vi "ttm_creep_poller.vi"() -> ()   [LabVIEW 2011]
doc: "This is the sample data playback waveform and data logging example program. Sample data points are generated using MX Sample Data Array Generator.vi. You will need to replace this VI with your own code. New sample data is sent to the controller each time a status message is recieved from the controller that the next random buffer is running.\nThis program also shows you how to use Active X events. These are used to notify the program when a data buffer is ready for collection and when to load a new buffer of sample data points. Two separate event queues are used: one for data logging and the other for general status, such as when a sample data point buffer can be sent to the controller. Each event handler must run in parallel loops as execution passes to MX Handle Status Change Event.vi and MX Handle Data Ready Event.vi and will not come out of them until an event is received from the console program. When modifiying this example for your own use you may want to setup a third loop to be doing other processing, or you could add code to manipulate the data buffer in the data monitoring loop."
panel:
  out "Number of points":i32=1000
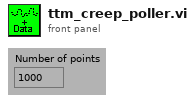
[diagram p1: front panel]
types:
  T1 = cluster{"Data Sample Format (0)":i8, "Loop code (2)":i8, "Target Amplitude (32767)":i16, "Playback rate":dbl, "Playback Scale":dbl[], "Envelope Ramp Rate":dbl, "Filter Order (0)":i8, "Filter Type (0)":i8, "Filter Bandwidth":dbl}
  T2 = cluster{"Name":string, "Type":i32, "SI Full Scale":dbl, "Full Scale":dbl, "Units String":string, "Display Format":string, "Gauge Length":dbl}[][]
  T3 = cluster{"Device ID":i32, "Device Name":string, "Device Type":i32}[]
  T4 = cluster{"Axis Information Out[0]":cluster{"Device ID":i32, "Device Name":string, "Device Type":i32}, "Axis Information Out[1]":cluster{"Device ID":i32, "Device Name":string, "Device Type":i32}, "Axis Information Out[2]":cluster{"Device ID":i32, "Device Name":string, "Device Type":i32}, "Axis Information Out[3]":cluster{"Device ID":i32, "Device Name":string, "Device Type":i32}, "Axis Information Out[4]":cluster{"Device ID":i32, "Device Name":string, "Device Type":i32}, "Axis Information Out[5]":cluster{"Device ID":i32, "Device Name":string, "Device Type":i32}, "Axis Information Out[6]":cluster{"Device ID":i32, "Device Name":string, "Device Type":i32}, "Axis Information Out[7]":cluster{"Device ID":i32, "Device Name":string, "Device Type":i32}, "Axis Information Out[8]":cluster{"Device ID":i32, "Device Name":string, "Device Type":i32}}
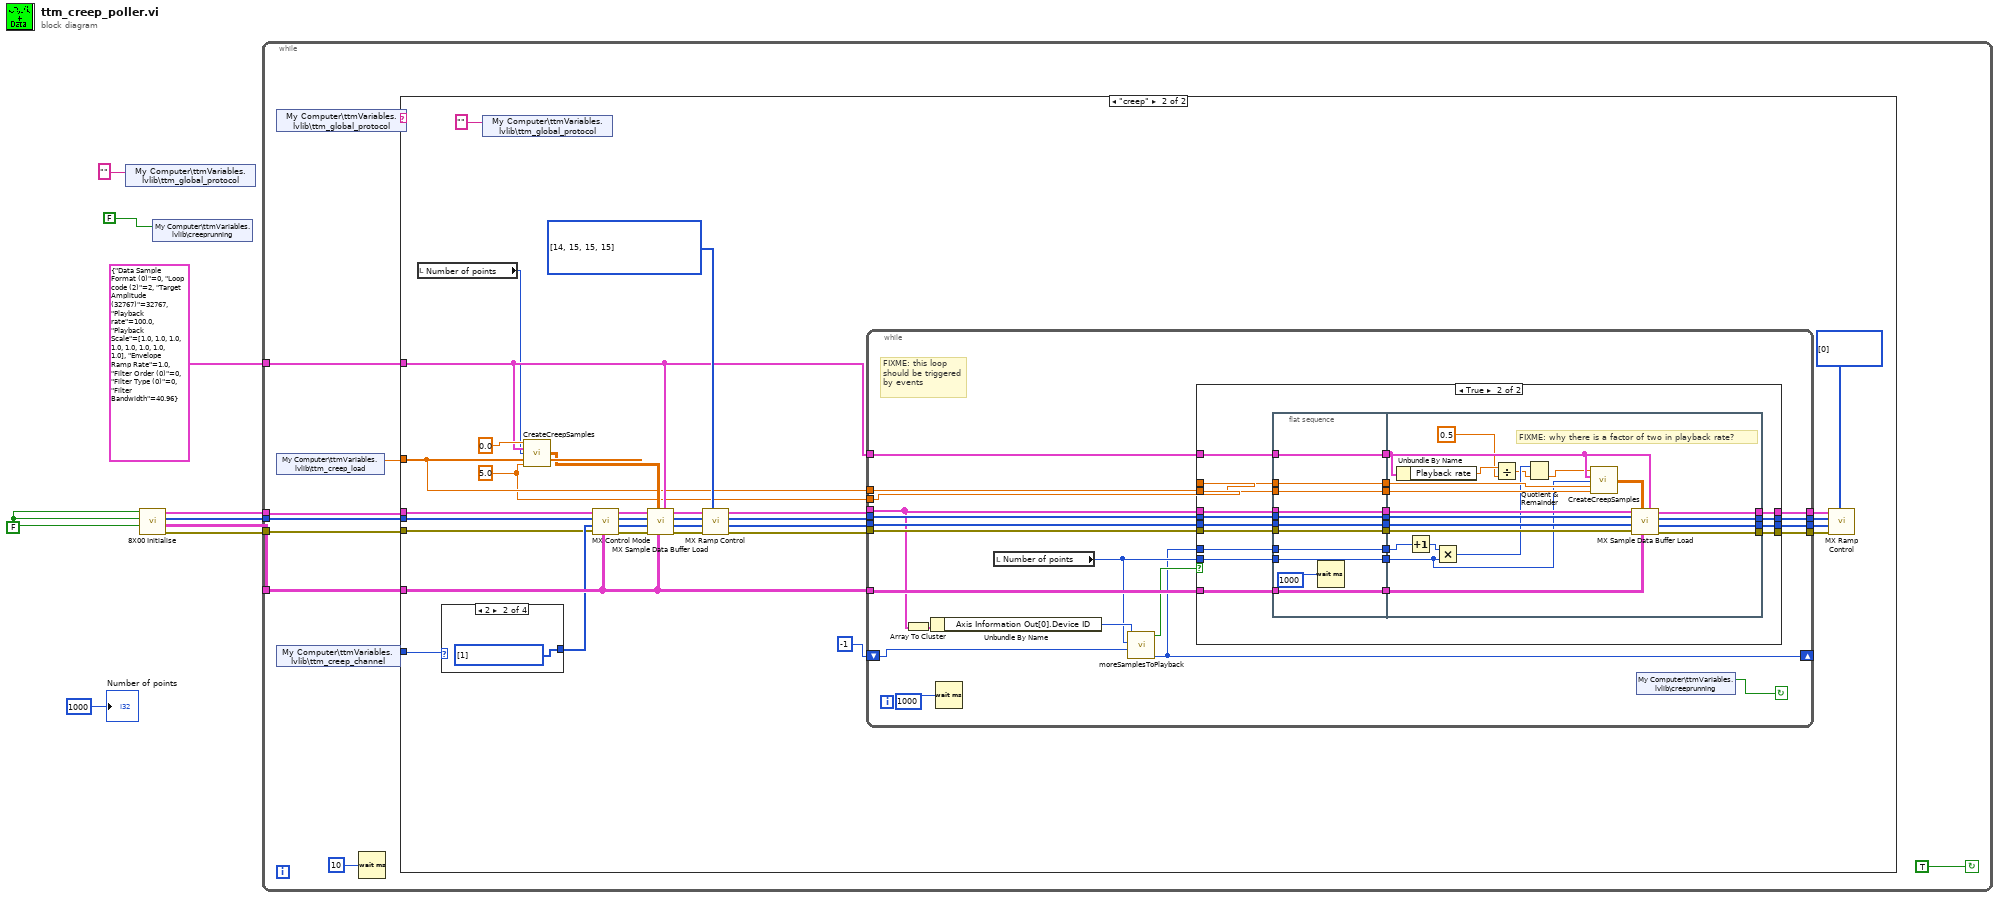
[diagram p0: block diagram]
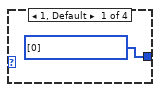
[diagram p3: hidden frame]
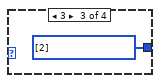
[diagram p4: hidden frame]
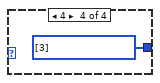
[diagram p5: hidden frame]
diagram:
  w6 = FALSE ("Reset")
  n1 = shared-variable "My Computer\\ttmVariables.lvlib\\ttm_global_protocol"("" ("protocol")) -> ()  [unwired: 1 in, 1 out]
  n2 = call "8X00 Initialise.vi"("Reset?"=w6, "Create DVM? (T)"=w6, "Create Console? (T)"=w6) -> ("error out"=w9:errorcluster, "Channel Data"=w8:T2, "Axis Selector"=w5:i32[], "Axis Information"=w7:T3)  [unwired: 1 in]
  n3 = shared-variable "My Computer\\ttmVariables.lvlib\\creeprunning"(FALSE ("startCreep")) -> ()  [unwired: 1 in, 1 out]
  n4 = while {
    tunnel: w8 -> [w19]
    tunnel: w7 -> [w15]
    tunnel: w9 -> [w13]
    tunnel: w5 -> [w14]
    tunnel: T1 {"Data Sample Format (0)"=0, "Loop code (2)"=2, "Target Amplitude (32767)"=32767, "Playback rate"=100.0, "Playback Scale"=[1.0, 1.0, 1.0, 1.0, 1.0, 1.0, 1.0, 1.0], "Envelope Ramp Rate"=1.0, "Filter Order (0)"=0, "Filter Type (0)"=0, "Filter Bandwidth"=40.96} ("Sample Data Playback Definition") -> [w11]
    stop <- TRUE continue-if-true
    n5 = shared-variable "My Computer\\ttmVariables.lvlib\\ttm_global_protocol"() -> (w10:string)  [unwired: 1 in, 1 out]
    n6 = shared-variable "My Computer\\ttmVariables.lvlib\\ttm_creep_load"() -> (w16:dbl)  [unwired: 1 in, 1 out]
    n7 = shared-variable "My Computer\\ttmVariables.lvlib\\ttm_creep_channel"() -> (w12:i32)  [unwired: 1 in, 1 out]
    n8 = Wait (ms)(milliseconds to wait=u32 10) -> ()  [unwired: 1 out]
    n9 = case shown="\"creep\"" w10 {
      tunnel: w19 -> [_ w40]
      tunnel: w16 -> [_ w27]
      tunnel: w15 -> [_ w35]
      tunnel: w14 -> [_ w34]
      tunnel: w13 -> [_ w32]
      tunnel: w12 -> [_ w46]
      tunnel: w11 -> [_ w30]
      frame "", Default {
      }
      frame "creep" {
        w26 = 5.0 ("rampTimeInSeconds")
        w41 = u16[] [0] items=["Stop", "Start or continue", "Hold", "Continue", "Return ramp to set level at fixed rate", "Reserved", "Reserved", "Start Random without demand hold", "Start Random with demand hold", "Prepare Random Start without demand hold", "Prepare Random Start with demand hold", "Unslave", "Reserved", "Reserved", "Start Sample Data Playback or Resume", "Prepare for Start of Sample Data", "Reserved", "Reserved", "Resume Playback", "Start an electromechanical frame return"] ("Ramp Control")
        w47 = u16[] [14, 15, 15, 15] items=["Stop", "Start or continue", "Hold", "Continue", "Return ramp to set level at fixed rate", "Reserved", "Reserved", "Start Random without demand hold", "Start Random with demand hold", "Prepare Random Start without demand hold", "Prepare Random Start with demand hold", "Unslave", "Reserved", "Reserved", "Start Sample Data Playback or Resume", "Prepare for Start of Sample Data", "Reserved", "Reserved", "Resume Playback"] ("Ramp Control")
        n10 = local read "Number of points"() -> (w29:i32)
        n11 = case shown="2" w46 {
          tunnel: [w52 w53 w54 w55] -> w33
          frame 1, Default {
            w52 = u16[] [0] items=["Channel 1", "Channel 2", "Channel 3", "Channel 4"] ("Choose channel to apply\nthe setpoint")
          }
          frame 2 {
            w53 = u16[] [1] items=["Channel 1", "Channel 2", "Channel 3", "Channel 4"] ("Choose channel to apply\nthe setpoint")
          }
          frame 3 {
            w54 = u16[] [2] items=["Channel 1", "Channel 2", "Channel 3", "Channel 4"] ("Choose channel to apply\nthe setpoint")
          }
          frame 4 {
            w55 = u16[] [3] items=["Channel 1", "Channel 2", "Channel 3", "Channel 4"] ("Choose channel to apply\nthe setpoint")
          }
        }
        n12 = shared-variable "My Computer\\ttmVariables.lvlib\\ttm_global_protocol"("" ("protocol")) -> ()  [unwired: 1 in, 1 out]
        n13 = call "CreateCreepSamples.vi"("t0"=0.0, "input cluster"=w30, "outputLength"=w29, "loadInNewtons"=w27, "rampTimeInSeconds"=w26) -> ("output array"=w28:dbl[][])  [unwired: 10 in]
        n14 = call "MX Control Mode.vi"("Channel Data"=w40, "error in (no error)"=w32, "Control Modes"=w33, "Axis Selector"=w34, "Axis Information"=w35) -> ("error out"=w36:errorcluster, "Control Modes out"=w37:u16[], "Axis Selector out"=w38:i32[], "Axis Information out"=w39:T3)  [unwired: 1 in]
        n15 = call "MX Sample Data Buffer Load.vi"("Sample Data Playback Definition"=w30, "Channel Data"=w40, "Sample Data"=w28, "error in (no error)"=w36, "Channels In"=w37, "Axis Selector In"=w38, "Axis Information In"=w39) -> ("error out"=w49:errorcluster, "Channels Out"=w48:u16[], "Axis Selector Out"=w50:i32[], "Axis Information Out"=w51:T3)  [unwired: 1 in]
        n16 = call "MX Ramp Control.vi"("Ramp Control"=w47, "error in (no error)"=w49, "Channels In"=w48, "Axis Selector In"=w50, "Axis Information In"=w51) -> ("error out"=w21:errorcluster, "Channels Out"=w22:u16[], "Axis Selector Out"=w23:i32[], "Axis Information Out"=w24:T3)  [unwired: 2 in]
        n17 = while {
          tunnel: w24 -> [w64]
          tunnel: w23 -> [w75]
          tunnel: w22 -> [w68]
          tunnel: w21 -> [w74]
          tunnel: [w65] -> w45
          tunnel: [w73] -> w44
          tunnel: [w72] -> w43
          tunnel: [w71] -> w42
          tunnel: w30 -> [w61]
          tunnel: w40 -> [w70]
          tunnel: w27 -> [w58]
          tunnel: w26 -> [w59]
          shift-right: [w56] -> _
          shift-left: -1 ("currentSampleCycle") -> [w60]
          stop <- w69 continue-if-true
          # "FIXME: this loop \nshould be triggered \nby events"
          n18 = Array To Cluster(array=w64) -> (cluster=w66:T4)
          n19 = Unbundle By Name(w66) -> ("Axis Information Out[0].Device ID"=w63:i32)
          n20 = Wait (ms)(milliseconds to wait=u32 1000) -> ()  [unwired: 1 out]
          n21 = local read "Number of points"() -> (w57:i32)
          n22 = call "moreSamplesToPlayback.vi"("Device"=w63, "playbackCycleLength"=w57, "previousSampleCycle"=w60) -> ("ReadyForMore"=w62:bool, "currentSampleCycle"=w56:i32)  [unwired: 6 in]
          n23 = case shown="True" w62 {
            tunnel: w75 -> [w78 w103]
            tunnel: w74 -> [w76 w102]
            tunnel: [w78 w101] -> w73
            tunnel: [w77 w100] -> w72
            tunnel: [w76 w99] -> w71
            tunnel: w61 -> [_ w90]
            tunnel: w70 -> [_ w98]
            tunnel: w68 -> [w77 w97]
            tunnel: [w79 w96] -> w65
            tunnel: w64 -> [w79 w95]
            tunnel: w59 -> [_ w94]
            tunnel: w58 -> [_ w93]
            tunnel: w57 -> [_ w91]
            tunnel: w56 -> [_ w92]
            frame False {
            }
            frame True {
              n24 = flat-sequence {
                tunnel: w90 -> [w105]
                tunnel: w91 -> [w106]
                tunnel: w92 -> [w107]
                tunnel: w93 -> [w108]
                tunnel: w94 -> [w109]
                tunnel: w95 -> [w110]
                tunnel: w97 -> [w111]
                tunnel: w98 -> [w112]
                tunnel: w102 -> [w113]
                tunnel: w103 -> [w114]
                tunnel: [w114] -> w89
                tunnel: [w113] -> w88
                tunnel: [w112] -> w87
                tunnel: [w111] -> w86
                tunnel: [w110] -> w85
                tunnel: [w109] -> w84
                tunnel: [w108] -> w83
                tunnel: [w107] -> w82
                tunnel: [w106] -> w81
                tunnel: [w105] -> w80
                tunnel: [w133] -> w101
                tunnel: [w132] -> w100
                tunnel: [w131] -> w99
                tunnel: [w128] -> w96
                tunnel: w89 -> [w135]
                tunnel: w88 -> [w134]
                tunnel: w87 -> [w130]
                tunnel: w86 -> [w129]
                tunnel: w85 -> [w127]
                tunnel: w84 -> [w125]
                tunnel: w83 -> [w124]
                tunnel: w82 -> [w115]
                tunnel: w81 -> [w123]
                tunnel: w80 -> [w122]
                frame #0 {
                  n25 = Wait (ms)(milliseconds to wait=u32 1000) -> ()  [unwired: 1 out]
                }
                frame #1 {
                  # "FIXME: why there is a factor of two in playback rate?"
                  n26 = Unbundle By Name(w122) -> ("Playback rate"=w119:dbl)
                  n27 = Increment(x=w115) -> (x+1=w116:i32)
                  n28 = Multiply(x=w116, y=w123) -> (x*y=w121:i32)
                  n29 = Divide(x=w119, y=0.5) -> (x/y=w118:dbl)
                  n30 = Quotient & Remainder(x=w121, y=w118) -> (floor(x/y)=w120:dbl)  [unwired: 1 out]
                  n31 = call "CreateCreepSamples.vi"("t0"=w120, "input cluster"=w122, "outputLength"=w123, "loadInNewtons"=w124, "rampTimeInSeconds"=w125) -> ("output array"=w126:dbl[][])  [unwired: 10 in]
                  n32 = call "MX Sample Data Buffer Load.vi"("Sample Data Playback Definition"=w122, "Channel Data"=w130, "Sample Data"=w126, "error in (no error)"=w134, "Channels In"=w129, "Axis Selector In"=w135, "Axis Information In"=w127) -> ("error out"=w131:errorcluster, "Channels Out"=w132:u16[], "Axis Selector Out"=w133:i32[], "Axis Information Out"=w128:T3)  [unwired: 1 in]
                }
              }
            }
          }
          n33 = shared-variable "My Computer\\ttmVariables.lvlib\\creeprunning"() -> (w69:bool)  [unwired: 1 in, 1 out]
        }
        n34 = call "MX Ramp Control.vi"("Ramp Control"=w41, "error in (no error)"=w42, "Channels In"=w43, "Axis Selector In"=w44, "Axis Information In"=w45) -> ()  [unwired: 2 in, 4 out]
      }
    }
  }
  "Number of points" <- 1000 ("Number of points")
